vi "XY Graph Try Plot Name.vi"(8 "Error In":errorcluster, 10 "Plot Name in":string, 11 "XY Graph Refnum":T1) -> (0 "Error Out":errorcluster, 2 "Plot Name out":string, 3 "XY Graph Refnum":T1, 5 "Graph Caption (or Label)":string)   [LabVIEW 2021, in "XY Graph Add-Ons.lvlib"]
uses:
  XY Graph Refnum.ctl
  XY Graph Add-Ons.lvlib
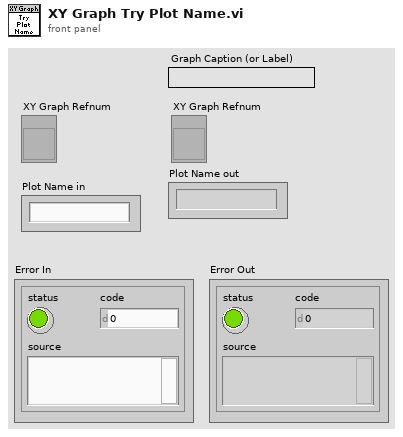
[diagram p1: front panel]
types:
  T1 = typedef "XY Graph Add-Ons.lvlib/XY Graph Refnum.ctl" = refnum<vi>
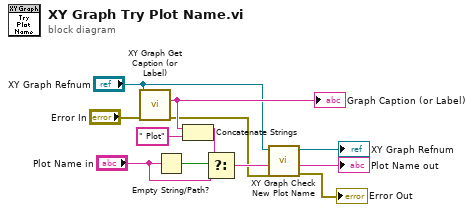
[diagram p0: block diagram]
diagram:
  n1 = call "XY Graph Get Caption (or Label).vi"("error in (no error)"="Error In", "XYGraph in"="XY Graph Refnum") -> ("error out"=w1:errorcluster, "Caption (or Label) Text"=w12:string)  [unwired: 7 in, 1 out]
  "Graph Caption (or Label)" <- w12
  n2 = Empty String/Path?(string/path="Plot Name in") -> (empty?=w10:bool)
  n3 = Concatenate Strings(w12, " Plot" ("string")) -> (w9:string)
  n4 = Select(t=w9, s=w10, f="Plot Name in") -> (s? t:f=w7:string)
  n5 = call "XY Graph Check New Plot Name.vi"("Error In"=w1, "New Plot Name (in)"=w7, "Multiplot XY Graph Refnum in"="XY Graph Refnum") -> ("Error Out"=→"Error Out":errorcluster, "New Plot Name (out)"=→"Plot Name out":string, "Multiplot XY Graph Refnum out"=→"XY Graph Refnum":T1)  [unwired: 6 in]
